vi "get_rumble_latest.vi"(8 "error in (no error)":errorcluster) -> (0 "error out":errorcluster, 2 "First-page median":cluster{"ID":i32, "Time":timestamp}, 3 "Latest":cluster{"ID":i32, "Time":timestamp})   [LabVIEW 2023]
uses:
  <vilib>/Analysis/NI_AALBase.lvlib
  <vilib>/httpClient/LabVIEWHTTPClient.lvlib
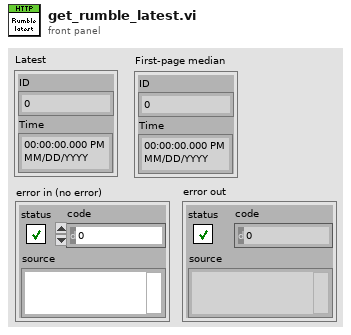
[diagram p1: front panel]
types:
  T1 = typedef "LabVIEWHTTPClient.lvlib/ClientHandle.ctl" = refnum<k1>
  T2 = cluster{"Title":string, "Channel":string, "Duration (s)":i32, "Is streaming":bool, "Timestamp":timestamp}
  T3 = cluster{"Video URL":string, "Video info":string, "HTTP result":i32}
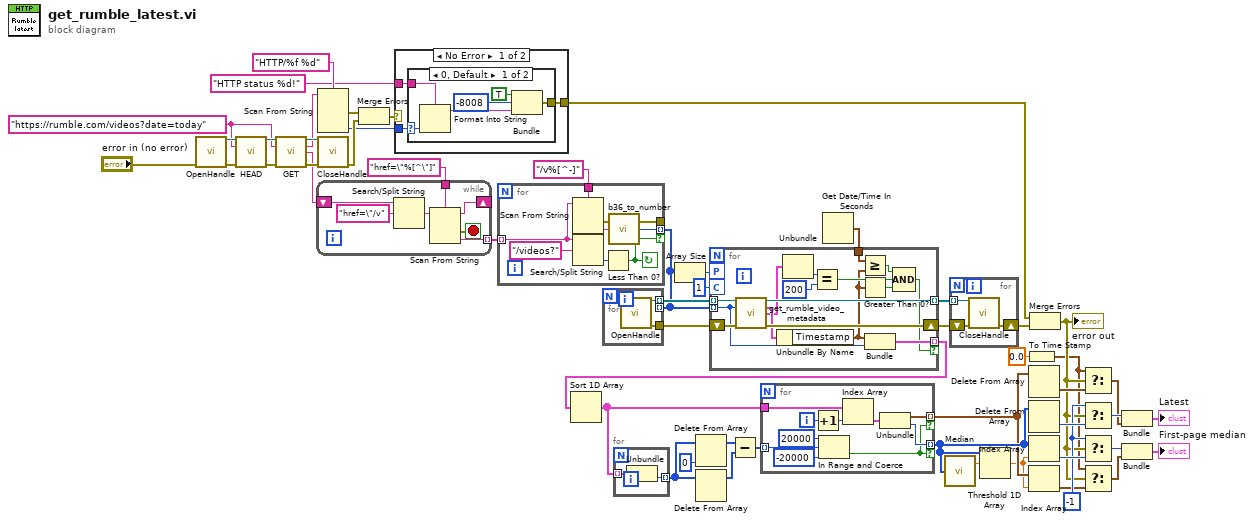
[diagram p0: block diagram]
diagram:
  w13 = -1 ("t")
  w45 = "https://rumble.com/videos?date=today"
  n1 = call <vilib>:"OpenHandle.vi"("error in (no error)"="error in (no error)") -> ("client handle out"=w49:T1, "error out"=w48:errorcluster)  [unwired: 13 in]
  n2 = call <vilib>:"HEAD.vi"("client handle"=w49, "url"=w45, "error in (no error)"=w48) -> ("client handle out"=w47:T1, "error out"=w46:errorcluster)  [unwired: 10 in, 1 out]
  n3 = call <vilib>:"GET.vi"("client handle"=w47, "url"=w45, "error in (no error)"=w46) -> ("client handle out"=w50:T1, "headers"=w41:string, "body"=w43:string, "error out"=w51:errorcluster)  [unwired: 9 in]
  n4 = while {
    shift-right: [w58] -> _
    shift-left: w43 -> [w61]
    tunnel: [w56] -> w53 mode=indexing
    tunnel: "href=\"%[^\"]" ("String") -> [w55]
    stop <- w57 stop-if-true
    n5 = Search/Split String(string=w61, search string/char (-)="href=\"/v" ("String")) -> (match + rest of string=w59:string)  [unwired: 1 in, 2 out]
    n6 = Scan From String(format string=w55, input string=w59) -> (remaining string=w58:string, error out=w57:errorcluster, output 1=w56:string)  [unwired: 3 in, 1 out]
  }
  n7 = Scan From String(format string="HTTP/%f %d", input string=w41) -> (error out=w40:errorcluster, output 2=w38:i32)  [unwired: 5 in, 2 out]
  n8 = call <vilib>:"CloseHandle.vi"("client handle"=w50, "error in (no error)"=w51) -> ("error out"=w39:errorcluster)  [unwired: 13 in]
  n9 = Merge Errors(w40, w39) -> (w37:errorcluster)
  n10 = case shown="No Error" w37 {
    selector: w37 -> [_ w71]
    tunnel: w38 -> [w64 _]
    tunnel: [w62 w71] -> w20
    tunnel: "HTTP status %d!" ("format string") -> [w63 _]
    frame No Error {
      n11 = case shown="0, Default" w64 {
        selector: w64 -> [w70 _]
        tunnel: w63 -> [w69 _]
        tunnel: [w65 _] -> w62
        frame 0, Default {
          n12 = Format Into String(format string=w69, w70) -> (resulting string=w68:string)  [unwired: 2 in, 1 out]
          n13 = Bundle("status"=TRUE, "code"=-8008, w68) -> (w65:cluster{"status":bool, "code":i32, string})  [unwired: 1 in]
        }
        frame 200 {
        }
      }
    }
    frame Error {
    }
  }
  n14 = for {
    tunnel: w53 -> [w76] mode=indexing
    tunnel: [w72] -> w7 mode=indexing if=w77
    tunnel: "/v%[^-]" ("String") -> [w75]
    tunnel: [w74] -> _
    stop <- w77 continue-if-true
    n15 = Scan From String(format string=w75, input string=w76) -> (error out=w74:errorcluster, output 1=w73:string)  [unwired: 3 in, 2 out]
    n16 = Search/Split String(string=w76, search string/char (-)="/videos?") -> (offset of match=w78:i32)  [unwired: 1 in, 2 out]
    n17 = Less Than 0?(x=w78) -> (x < 0?=w77:bool)
    n18 = call "b36_to_number.vi"("Base36 string"=w73) -> ("Number"=w72:i32)
  }
  n19 = for {
    tunnel: [w81] -> w34 mode=indexing
    tunnel: [w80] -> w32
    tunnel: w7 -> [_] mode=indexing
    n20 = call <vilib>:"OpenHandle.vi"() -> ("client handle out"=w81:T1, "error out"=w80:errorcluster)  [unwired: 14 in]
  }
  n21 = Array Size(array=w7) -> (size(s)=w33:i32)
  n22 = Get Date/Time In Seconds() -> (seconds since 1Jan1904=w25:timestamp)
  n23 = for {
    shift-right: [w96] -> w30
    shift-left: w32 -> [w97]
    tunnel: w7 -> [w94] mode=indexing
    tunnel: [w93] -> w22 mode=indexing if=w88
    workers-P: w33 -> [_]
    chunk-C: 1 -> [_]
    tunnel: w34 -> [w92] mode=indexing
    tunnel: [w91] -> w31 mode=indexing
    tunnel: w25 -> [w85]
    n24 = call "get_rumble_video_metadata.vi"("HTTP client handle"=w92, "Video ID"=w94, "error in (no error)"=w97) -> ("client handle out"=w91:T1, "Video data"=w95:T2, "Query result"=w83:T3, "error out"=w96:errorcluster)  [unwired: 8 in, 1 out]
    n25 = Unbundle By Name(w95) -> ("Timestamp"=w86:timestamp)
    n26 = Unbundle(w83) -> ("HTTP result"=w82:i32)  [unwired: 2 out]
    n27 = Equal?(x=w82, y=200 ("x")) -> (x = y?=w89:bool)
    n28 = Greater Or Equal?(x=w85, y=w86) -> (x >= y?=w84:bool)
    n29 = Greater Than 0?(x=w86) -> (x > 0?=w87:bool)
    n30 = Bundle("Timestamp"=w86, "Number"=w94) -> (w93:cluster{"Timestamp":timestamp, "Number":i32})  [unwired: 1 in]
    n31 = Compound Arithmetic op=AND(w84, w89, w87) -> (w88:bool)
  }
  n32 = Sort 1D Array(array=w22) -> (sorted array=w23:cluster{"Timestamp":timestamp, "Number":i32}[])
  n33 = for {
    tunnel: w23 -> [w99] mode=indexing
    tunnel: [w98] -> w29 mode=indexing
    n34 = Unbundle(w99) -> ("Number"=w98:i32)  [unwired: 1 out]
  }
  n35 = Delete From Array(array=w29, index=0) -> (array with subset deleted=w27:i32[])  [unwired: 1 in, 1 out]
  n36 = Delete From Array(array=w29) -> (array with subset deleted=w26:i32[])  [unwired: 2 in, 1 out]
  n37 = Subtract(x=w27, y=w26) -> (x-y=w24:i32[])
  n38 = for {
    tunnel: w24 -> [w109] mode=indexing
    tunnel: [w102] -> w16 mode=indexing if=w100
    tunnel: w23 -> [w105]
    tunnel: [w101] -> w15 mode=indexing if=w100
    i -> [w106]
    n39 = Increment(x=w106) -> (x+1=w104:i32)
    n40 = In Range and Coerce(upper limit=20000, x=w109, lower limit=-20000) -> (In Range?=w100:bool)  [unwired: 1 out]
    n41 = Index Array(array=w105, index=w104) -> (element=w103:cluster{"Timestamp":timestamp, "Number":i32})
    n42 = Unbundle(w103) -> ("Timestamp"=w101:timestamp, "Number"=w102:i32)
  }
  n43 = call <vilib>:"Median.vi"("X"=w16) -> ("median"=w17:dbl)  [unwired: 1 out]
  n44 = for {
    tunnel: w31 -> [w112] mode=indexing
    shift-right: [w110] -> w21
    shift-left: w30 -> [w111]
    n45 = call <vilib>:"CloseHandle.vi"("client handle"=w112, "error in (no error)"=w111) -> ("error out"=w110:errorcluster)  [unwired: 13 in]
  }
  n46 = Threshold 1D Array(2:w17, 3:w16) -> (0:w14:dbl)  [unwired: 1 in]
  n47 = To Time Stamp(1:0.0 ("number")) -> (0:w8:timestamp)
  n48 = Delete From Array(array=w15) -> (deleted portion=w12:timestamp)  [unwired: 2 in, 1 out]
  n49 = Delete From Array(array=w16) -> (deleted portion=w18:i32)  [unwired: 2 in, 1 out]
  n50 = Index Array(array=w16, index=w14) -> (element=w19:i32)
  n51 = Index Array(array=w15, index=w14) -> (element=w10:timestamp)
  n52 = Merge Errors(w20, w21) -> (w9:errorcluster)
  "error out" <- w9
  n53 = Select(t=w8, s=w9, f=w12) -> (s? t:f=w5:timestamp)
  n54 = Select(t=w13, s=w9, f=w18) -> (s? t:f=w6:i32)
  n55 = Select(t=w13, s=w9, f=w19) -> (s? t:f=w4:i32)
  n56 = Select(t=w8, s=w9, f=w10) -> (s? t:f=w3:timestamp)
  n57 = Bundle("Number"=w6, "Timestamp"=w5) -> (→"Latest":cluster{"Number":i32, "Timestamp":timestamp})  [unwired: 1 in]
  n58 = Bundle("Number"=w4, "Timestamp"=w3) -> (→"First-page median":cluster{"Number":i32, "Timestamp":timestamp})  [unwired: 1 in]
